vi "LPCA Command Builder.vi"(8 "error in (no error)":errorcluster, 9 "Data":string, 10 "LPCA Command":T1, 11 "Mode":enum16{"set", "query"}(ring)) -> (0 "error out":errorcluster, 3 "String":string)   [LabVIEW 2017]
uses:
  Controls/LPCA Commands.ctl
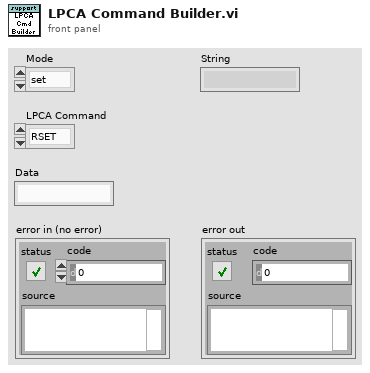
[diagram p1: front panel]
types:
  T1 = typedef "LPCA Commands.ctl" = enum16{"RSET", "stop", "rpmh", "rpml", "prpm", "rpm", "mamp", "rng", "tmp1", "tmp2", "err", "ramp"}
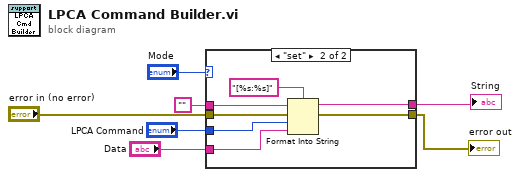
[diagram p0: block diagram]
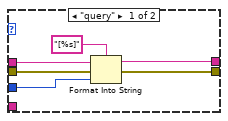
[diagram p2: hidden frame]
diagram:
  n1 = case shown="\"set\"" "Mode" {
    tunnel: "LPCA Command" -> [w13 w20]
    tunnel: "" -> [w12 w19]
    tunnel: [w10 w17] -> w7
    tunnel: "Data" -> [_ w16]
    tunnel: "error in (no error)" -> [w8 w15]
    tunnel: [w9 w14] -> w6
    frame "query" {
      n2 = Format Into String(format string="[%s]", initial string=w12, error in=w8, w13) -> (resulting string=w10:string, error out=w9:errorcluster)
    }
    frame "set" {
      n3 = Format Into String(format string="[%s:%s]", initial string=w19, error in=w15, w20, w16) -> (resulting string=w17:string, error out=w14:errorcluster)
    }
  }
  "String" <- w7
  "error out" <- w6
